vi "addReportServerStatusFrame.vi"(8 "error in (no error)":errorcluster, 10 "ModbusBuffer in":refnum<class "ModbusBuffer.lvclass">, 11 "ILC in":refnum<class "ILC.lvclass">) -> (0 "error out":errorcluster, 2 "ModbusBuffer out":refnum<class "ModbusBuffer.lvclass">, 3 "ILC out":refnum<class "ILC.lvclass">)   [LabVIEW 2016, in "RTILC.lvlib" / "ILC.lvclass"]
uses:
  ILC.lvclass
  Common_RT_Modbus/ModbusBuffer/ModbusBuffer.lvclass
  ILC.lvclass/ILC.ctl
  Common_RT_Modbus/DataTypes/ExceptionCodes.ctl
  Common_RT_Modbus/ModbusBuffer/ModbusBuffer.lvclass/ModbusBuffer.ctl
  Common_RT_Modbus/ModbusBuffer/writeByteInstruction.vi
  Common_RT_Modbus/ModbusBuffer/calculateCRC.vi
  Common_RT_Modbus/RTModbus.lvlib
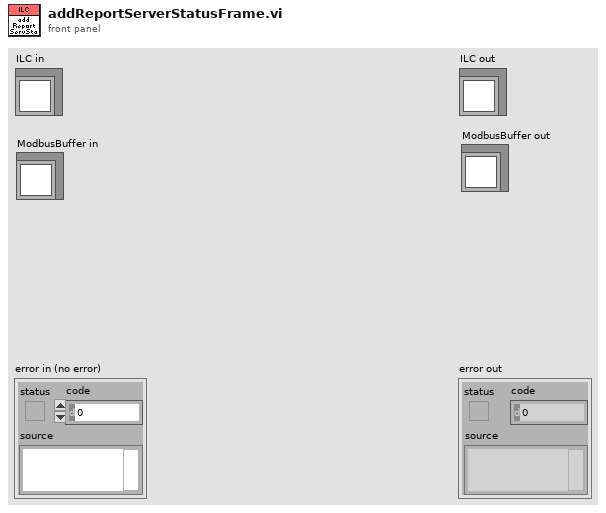
[diagram p1: front panel]
types:
  T1 = typedef "RTModbus.lvlib/ExceptionCodes.ctl" = u16
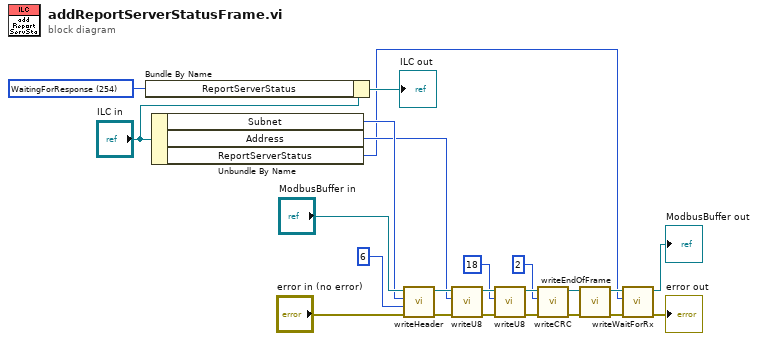
[diagram p0: block diagram]
diagram:
  w23 = T1 254 items=["OK"=0, "IllegalFunction"=1, "IllegalDataAddress"=2, "IllegalDataValue"=3, "SlaveDeviceFailure"=4, "Acknowledge"=5, "SlaveDeviceBusy"=6, "NegativeAcknowledge"=7, "MemoryParityError"=8, "GatewayPathUnavailable"=9, "GatewayTargetDeviceFailedToRespond"=10, "WaitingForResponse"=254, "CRCError"=255] ("ILCData.Responses.ADCOffsetSensitivity")
  n1 = Bundle By Name(cluster="ILC in", "ReportServerStatus"=w23) -> (→"ILC out":refnum<class "ILC.lvclass">)
  n2 = Unbundle By Name("ILC in") -> ("Subnet"=w6:u8, "Address"=w4:u8, "ReportServerStatus"=w1:u32)
  n3 = call "writeHeader.vi"("error in (no error)"="error in (no error)", "Length"=u16 6, "Subnet"=w6, "ModbusBuffer in"="ModbusBuffer in") -> ("error out"=w12:errorcluster, "ModbusBuffer out"=w19:refnum<class "ModbusBuffer.lvclass">)  [unwired: 6 in]
  n4 = call "writeU8.vi"("error in (no error)"=w12, "Input"=w4, "ModbusBuffer in"=w19) -> ("error out"=w11:errorcluster, "ModbusBuffer out"=w18:refnum<class "ModbusBuffer.lvclass">)  [unwired: 7 in]
  n5 = call "writeU8.vi"("error in (no error)"=w11, "Input"=u8 18 ("Byte"), "ModbusBuffer in"=w18) -> ("error out"=w10:errorcluster, "ModbusBuffer out"=w17:refnum<class "ModbusBuffer.lvclass">)  [unwired: 7 in]
  n6 = call "writeCRC.vi"("error in (no error)"=w10, "Length"=2, "ModbusBuffer in"=w17) -> ("error out"=w9:errorcluster, "ModbusBuffer out"=w16:refnum<class "ModbusBuffer.lvclass">)  [unwired: 7 in]
  n7 = call "writeEndOfFrame.vi"("error in (no error)"=w9, "ModbusBuffer in"=w16) -> ("error out"=w8:errorcluster, "ModbusBuffer out"=w15:refnum<class "ModbusBuffer.lvclass">)  [unwired: 8 in]
  n8 = call "writeWaitForRx.vi"("error in (no error)"=w8, "Timeout(us)"=w1, "ModbusBuffer in"=w15) -> ("error out"=→"error out":errorcluster, "ModbusBuffer out"=→"ModbusBuffer out":refnum<class "ModbusBuffer.lvclass">)  [unwired: 7 in]
